vi "GraphMain.vi"() -> ()   [LabVIEW 2009]
uses:
  GraphNode/GraphNode.lvclass
  Graph.lvclass
  position.ctl
  InsertSearch.ctl
  GraphSearch/GraphSearch.lvclass
  GraphSearch/method.ctl
panel:
  out "ignored":bool
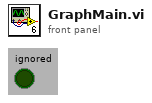
[diagram p1: front panel]
types:
  T1 = typedef "GraphSearch.lvclass/method.ctl" = enum16{"Breadth", "Heuristic", "Depth"}
  T2 = typedef "Graph.lvclass/InsertSearch.ctl" = cluster{"GraphSearch":refnum<class "GraphSearch.lvclass">, "InsertIfEmpty":bool}
  T3 = typedef "Graph.lvclass/position.ctl" = enum16{"Link To All", "Search"}
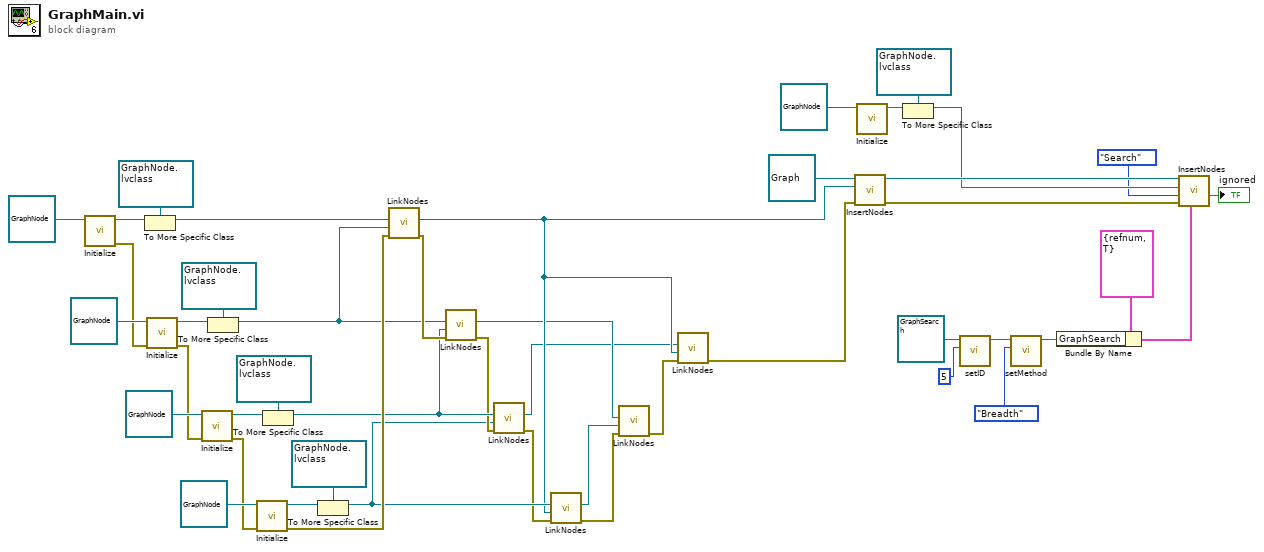
[diagram p0: block diagram]
diagram:
  n1 = call-dynamic "Initialize.vi"("GraphNode data"=refnum<class "GraphNode.lvclass"> refnum ("GraphNode.lvclass")) -> ("error out"=w40:errorcluster, "Node out"=w43:refnum<data-value>)  [unwired: 9 in]
  n2 = To More Specific Class(target class=refnum<data-value> refnum ("data value reference"), reference=w43) -> (specific class reference=w31:refnum<data-value>)  [unwired: 1 in, 1 out]
  n3 = call-dynamic "Initialize.vi"("error in (no error)"=w40, "GraphNode data"=refnum<class "GraphNode.lvclass"> refnum ("GraphNode.lvclass")) -> ("error out"=w36:errorcluster, "Node out"=w41:refnum<data-value>)  [unwired: 8 in]
  n4 = call-dynamic "Initialize.vi"("error in (no error)"=w36, "GraphNode data"=refnum<class "GraphNode.lvclass"> refnum ("GraphNode.lvclass")) -> ("error out"=w32:errorcluster, "Node out"=w39:refnum<data-value>)  [unwired: 8 in]
  n5 = To More Specific Class(target class=refnum<data-value> refnum ("data value reference"), reference=w41) -> (specific class reference=w28:refnum<data-value>)  [unwired: 1 in, 1 out]
  n6 = call-dynamic "Initialize.vi"("error in (no error)"=w32, "GraphNode data"=refnum<class "GraphNode.lvclass"> refnum ("GraphNode.lvclass")) -> ("error out"=w30:errorcluster, "Node out"=w33:refnum<data-value>)  [unwired: 8 in]
  n7 = To More Specific Class(target class=refnum<data-value> refnum ("data value reference"), reference=w39) -> (specific class reference=w27:refnum<data-value>)  [unwired: 1 in, 1 out]
  n8 = To More Specific Class(target class=refnum<data-value> refnum ("data value reference"), reference=w33) -> (specific class reference=w25:refnum<data-value>)  [unwired: 1 in, 1 out]
  n9 = call "LinkNodes.vi"("error in (no error)"=w30, "GraphNode2 in"=w28, "GraphNode1 in"=w31) -> ("error out"=w29:errorcluster, "GraphNode1 out"=w19:refnum<data-value>)  [unwired: 6 in, 1 out]
  n10 = call "LinkNodes.vi"("error in (no error)"=w29, "GraphNode2 in"=w27, "GraphNode1 in"=w28) -> ("error out"=w26:errorcluster, "GraphNode1 out"=w18:refnum<data-value>)  [unwired: 6 in, 1 out]
  n11 = call "LinkNodes.vi"("error in (no error)"=w26, "GraphNode2 in"=w25, "GraphNode1 in"=w27) -> ("error out"=w24:errorcluster, "GraphNode1 out"=w17:refnum<data-value>)  [unwired: 6 in, 1 out]
  n12 = call "LinkNodes.vi"("error in (no error)"=w24, "GraphNode2 in"=w19, "GraphNode1 in"=w25) -> ("error out"=w23:errorcluster, "GraphNode1 out"=w16:refnum<data-value>)  [unwired: 6 in, 1 out]
  n13 = call "LinkNodes.vi"("error in (no error)"=w23, "GraphNode2 in"=w16, "GraphNode1 in"=w18) -> ("error out"=w22:errorcluster)  [unwired: 6 in, 2 out]
  n14 = call "LinkNodes.vi"("error in (no error)"=w22, "GraphNode2 in"=w19, "GraphNode1 in"=w17) -> ("error out"=w20:errorcluster)  [unwired: 6 in, 2 out]
  n15 = call "InsertNodes.vi"("error in (no error)"=w20, "ToInsert"=w19, "Graph in"=refnum<class "Graph.lvclass"> refnum ("Graph.lvclass")) -> ("error out"=w11:errorcluster, "Graph out"=w15:refnum<class "Graph.lvclass">)  [unwired: 6 in, 1 out]
  n16 = call-dynamic "Initialize.vi"("GraphNode data"=refnum<class "GraphNode.lvclass"> refnum ("GraphNode.lvclass")) -> ("Node out"=w12:refnum<data-value>)  [unwired: 9 in, 1 out]
  n17 = To More Specific Class(target class=refnum<data-value> refnum ("data value reference"), reference=w12) -> (specific class reference=w10:refnum<data-value>)  [unwired: 1 in, 1 out]
  n18 = call "setID.vi"("ID"=u32 5, "GraphSearch in"=refnum<class "GraphSearch.lvclass"> refnum ("GraphSearch.lvclass")) -> ("GraphSearch out"=w3:refnum<class "GraphSearch.lvclass">)  [unwired: 8 in, 1 out]
  n19 = call "setMethod.vi"("method"=method."Breadth", "GraphSearch in"=w3) -> ("GraphSearch out"=w2:refnum<class "GraphSearch.lvclass">)  [unwired: 8 in, 1 out]
  n20 = Bundle By Name(cluster=T2 {"GraphSearch"=refnum, "InsertIfEmpty"=TRUE} ("InsertSearch"), "GraphSearch"=w2) -> (w5:T2)
  n21 = call "InsertNodes.vi"("InsertSearch"=w5, "error in (no error)"=w11, "position"=position."Search", "ToInsert"=w10, "Graph in"=w15) -> ("ignored"=→"ignored":bool)  [unwired: 4 in, 2 out]
